vi "move template project.vi"(8 "error in (no error)":errorcluster, 10 "Path":path, 11 "NIVS_ScriptedModuleTemplate_MetaDataObj in":refnum<class "NIVS_ScriptedModuleTemplate_MetaDataObj.lvclass">) -> (0 "error out":errorcluster)   [LabVIEW 2014, in "NIVS_ScriptedModuleTemplate_MetaDataObj.lvclass"]
uses:
  NIVS_ScriptedModuleTemplate_MetaDataObj.lvclass
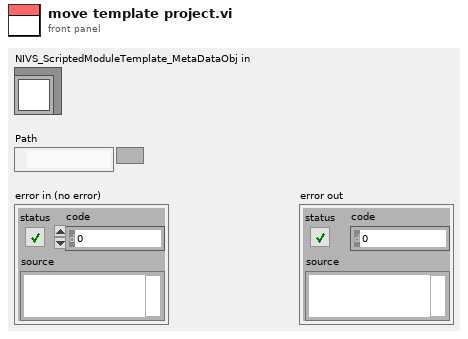
[diagram p1: front panel]
types:
  T1 = enum16{"open", "replace", "create", "open or create", "replace or create", "replace or create with confirmation"}
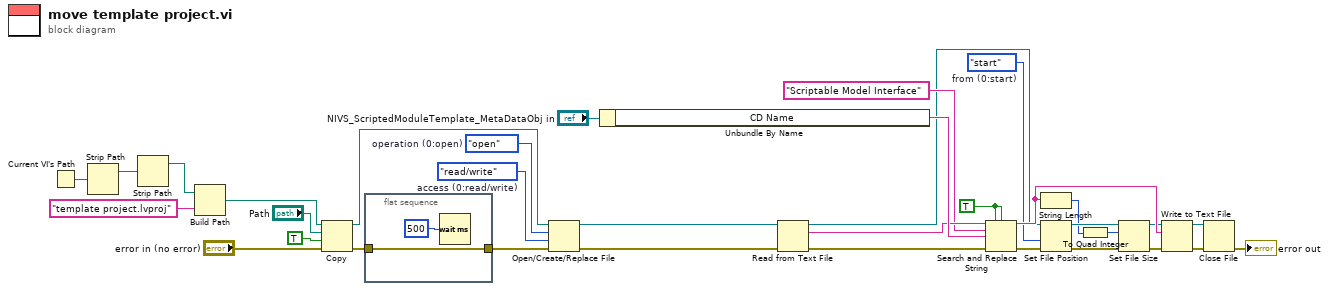
[diagram p0: block diagram]
diagram:
  w12 = enum16{"start", "end", "current"}."start"  # from (0:start)
  w19 = TRUE ("replace all? (F)")
  w23 = T1."open"  # operation (0:open)
  w24 = enum16{"read/write", "read-only", "write-only"}."read/write"  # access (0:read/write)
  n1 = Current VI's Path() -> (path=w1:path)
  n2 = Strip Path(path=w1) -> (stripped path=w2:path)  [unwired: 1 out]
  n3 = Strip Path(path=w2) -> (stripped path=w3:path)  [unwired: 1 out]
  n4 = Build Path(base path=w3, name or relative path="template project.lvproj") -> (appended path=w30:path)
  n5 = Copy(8:"error in (no error)", 9:TRUE ("overwrite (F)"), 10:"Path", 11:w30) -> (0:w33:errorcluster, 3:w32:path)  [unwired: 1 in, 1 out]
  n6 = flat-sequence {
    tunnel: w33 -> [w36]
    tunnel: [w36] -> w34
    frame #0 {
      n7 = Wait (ms)(milliseconds to wait=u32 500) -> ()  [unwired: 1 out]
    }
  }
  n8 = Open/Create/Replace File(file path (use dialog)=w32, error in=w34, operation (0:open)=w23, access (0:read/write)=w24) -> (refnum out=w26:refnum<file>, error out=w25:errorcluster)  [unwired: 3 out]
  n9 = Unbundle By Name("NIVS_ScriptedModuleTemplate_MetaDataObj in") -> ("CD Name"=w29:string)
  n10 = Read from Text File(file (use dialog)=w26, error in=w25) -> (refnum out=w9:refnum<file>, text=w22:string, error out=w21:errorcluster)  [unwired: 3 out]
  n11 = Search and Replace String(replace all?=w19, case sensitive?=w19, input string=w22, search string="Scriptable Model Interface", replace string=w29, error in=w21) -> (result string=w27:string, error out=w8:errorcluster)  [unwired: 2 in, 2 out]
  n12 = String Length(string=w27) -> (length=w11:i32)
  n13 = Set File Position(refnum=w9, from (0:start)=w12, error in=w8) -> (refnum out=w13:refnum<file>, error out=w14:errorcluster)  [unwired: 1 out]
  n14 = To Quad Integer(1:w11) -> (0:w10:i64)
  n15 = Set File Size(4:w14, 6:w10, 7:w13) -> (0:w16:errorcluster, 3:w15:refnum<file>)
  n16 = Write to Text File(file (use dialog)=w15, text=w27, error in=w16) -> (refnum out=w18:refnum<file>, error out=w17:errorcluster)  [unwired: 2 out]
  n17 = Close File(refnum=w18, error in=w17) -> (error out=→"error out":errorcluster)  [unwired: 1 out]
